vi "Add NI-XNET CAN Hardware_Add Incoming Single Point.vi"(6 "Single Point Frames":T1[](array[typedef]), 8 "error in (no error)":errorcluster, 9 "ClusterName":string, 10 "Owning Database":refnum<k24>, 11 "CAN Port":refnum<k24>) -> (0 "error out":errorcluster, 3 "CAN Port out":refnum<k24>)   [LabVIEW 2019, in "Simple SysDef API.lvlib"]
uses:
  <userlib>/SimpleSysDef/Simple SysDef API.lvlib
  <userlib>/SimpleSysDef/_SubVIs/Add NI-XNET CAN Hardware_Frame Settings.ctl
  <userlib>/SimpleSysDef/_SubVIs/Add NI-XNET CAN Hardware_Signal Settings.ctl
  NationalInstruments.VeriStand.SystemDefinitionAPI
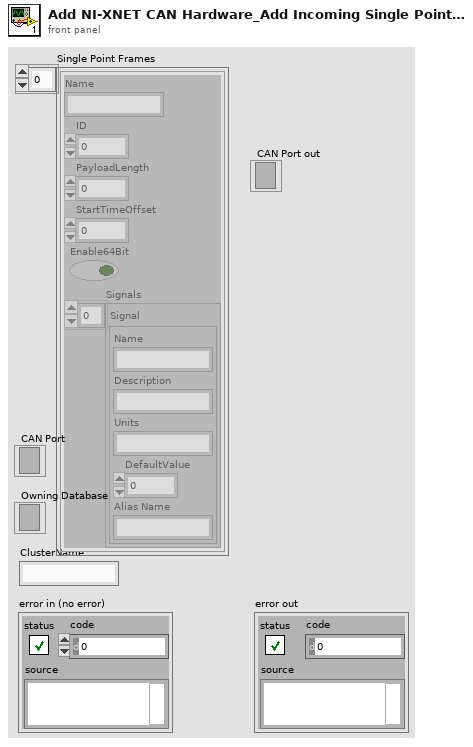
[diagram p1: front panel]
types:
  T1 = typedef "Simple SysDef API.lvlib/Add NI-XNET CAN Hardware_Frame Settings.ctl" = cluster{"Name":string, "ID":u32, "PayloadLength":u32, "StartTimeOffset":dbl, "Enable64Bit":bool, "Signals":T2[]}
  T2 = typedef "Simple SysDef API.lvlib/Add NI-XNET CAN Hardware_Signal Settings.ctl" = cluster{"Name":string, "Description":string, "Units":string, "DefaultValue":dbl, "Alias Name":string}
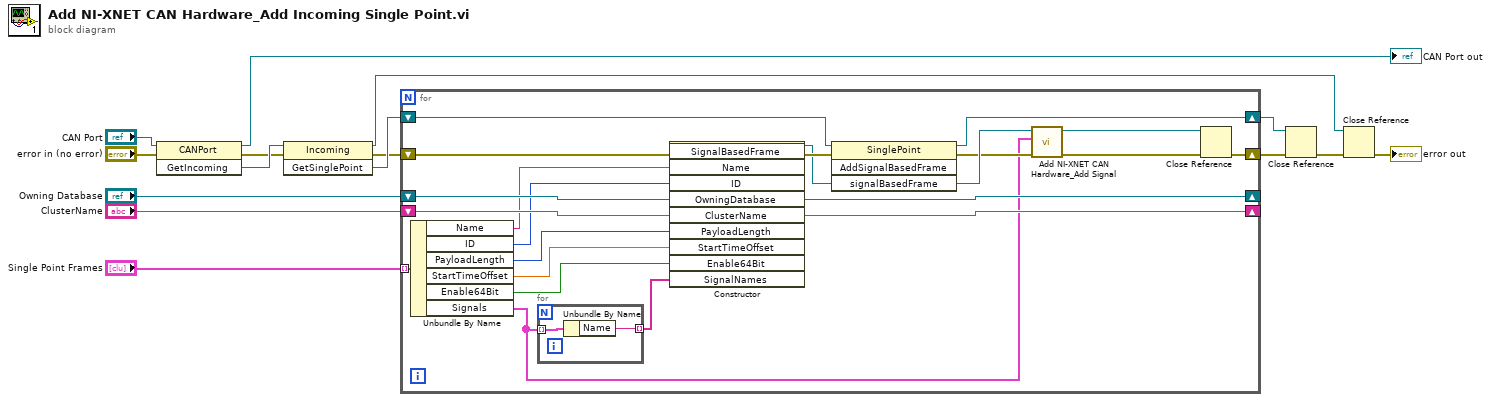
[diagram p0: block diagram]
diagram:
  n1 = invoke class="CANPort" method="GetIncoming"(reference="CAN Port", error in="error in (no error)") -> (reference out=→"CAN Port out":refnum<k24>, error out=w6:errorcluster, "GetIncoming"=w7:refnum<k24>)  [unwired: 1 in]
  n2 = invoke class="Incoming" method="GetSinglePoint"(reference=w7, error in=w6) -> (reference out=w1:refnum<k24>, error out=w11:errorcluster, "GetSinglePoint"=w12:refnum<k24>)  [unwired: 1 in]
  n3 = for {
    shift-right: [w31] -> _
    shift-left: "Owning Database" -> [w31]
    shift-right: [w30] -> _
    shift-left: "ClusterName" -> [w30]
    shift-right: [w28] -> w9
    shift-left: w11 -> [w33]
    shift-right: [w29] -> w10
    shift-left: w12 -> [w32]
    tunnel: "Single Point Frames" -> [w27] mode=indexing
    n4 = Unbundle By Name(w27) -> ("Name"=w26:string, "ID"=w25:u32, "PayloadLength"=w24:u32, "StartTimeOffset"=w23:dbl, "Enable64Bit"=w22:bool, "Signals"=w16:T2[])
    n5 = for {
      tunnel: w16 -> [w36] mode=indexing
      tunnel: [w35] -> w21 mode=indexing
      n6 = Unbundle By Name(w36) -> ("Name"=w35:string)
    }
    n7 = constructor class="SignalBasedFrame"(error in=w33, "Name"=w26, "ID"=w25, "OwningDatabase"=w31, "ClusterName"=w30, "PayloadLength"=w24, "StartTimeOffset"=w23, "Enable64Bit"=w22, "SignalNames"=w21) -> (reference out=w20:refnum<k24>, error out=w34:errorcluster)  [unwired: 2 in, 9 out]
    n8 = invoke class="SinglePoint" method="AddSignalBasedFrame"(reference=w32, error in=w34, "signalBasedFrame"=w20) -> (reference out=w29:refnum<k24>, error out=w18:errorcluster)  [unwired: 1 in, 2 out]
    n9 = call <userlib>:"Add NI-XNET CAN Hardware_Add Signal.vi"("error in (no error)"=w18, "Signals"=w16, "Frame Ref"=w20) -> ("error out"=w17:errorcluster, "Frame Ref out"=w19:refnum<k24>)  [unwired: 7 in]
    n10 = Close Reference(reference=w19, error in (no error)=w17) -> (error out=w28:errorcluster)
  }
  n11 = Close Reference(reference=w10, error in (no error)=w9) -> (error out=w3:errorcluster)
  n12 = Close Reference(reference=w1, error in (no error)=w3) -> (error out=→"error out":errorcluster)
